vi "MakeToAmbientCode.vi"(4 "ControlInput":string, 10 "AmbientTolerance":dbl=5.0, 11 "TAmbient":dbl=20.0 min=0.0 max=30.0) -> (3 "ToAmbient":string="define onecycle (pwm=100 run pwmloop 5A.PID.Setpoint=-131.500000  while(#3C >-129.5){pause 0.2 s}pwm=10 pause 10 min kill pwmloop pwm=0 relays=0 5A.PID.SetPoint=51.0 while(#3C<50.0){pause 0.2 s} pause 10 min)")   [LabVIEW 2024]
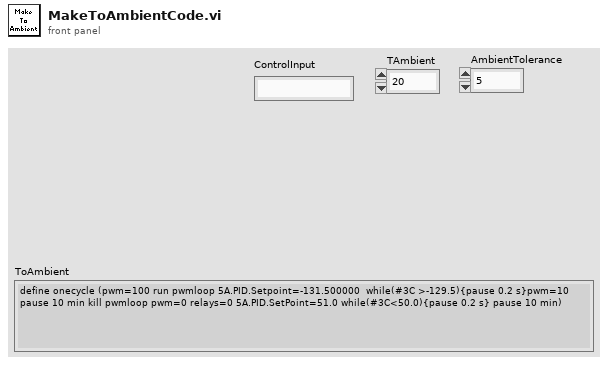
[diagram p1: front panel]
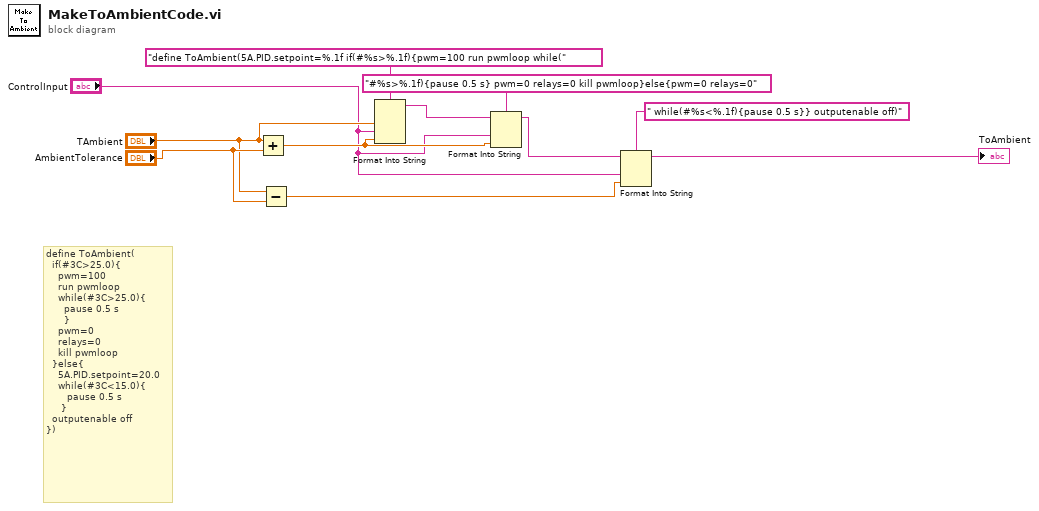
[diagram p0: block diagram]
diagram:
  # "define ToAmbient(\n  if(#3C>25.0){\n    pwm=100 \n    run pwmloop \n    while(#3C>25.0){\n      pause 0.5 s\n      } \n    pwm=0\n    relays=0 \n    kill pwmloop\n  }else{\n    5A.PID.setpoint=20.0 \n    while(#3C<15.0){\n       pause 0.5 s\n     } \n  outputenable off\n})"
  n1 = Add(x="TAmbient", y="AmbientTolerance") -> (x+y=w2:dbl)
  n2 = Subtract(x="TAmbient", y="AmbientTolerance") -> (x-y=w4:dbl)
  n3 = Format Into String(format string="define ToAmbient(5A.PID.setpoint=%.1f if(#%s>%.1f){pwm=100 run pwmloop while(", "TAmbient", "ControlInput", w2) -> (resulting string=w10:string)  [unwired: 2 in, 1 out]
  n4 = Format Into String(format string="#%s>%.1f){pause 0.5 s} pwm=0 relays=0 kill pwmloop}else{pwm=0 relays=0", initial string=w10, "ControlInput", w2) -> (resulting string=w7:string)  [unwired: 1 in, 1 out]
  n5 = Format Into String(format string=" while(#%s<%.1f){pause 0.5 s}} outputenable off)", initial string=w7, "ControlInput", w4) -> (resulting string=→"ToAmbient":string)  [unwired: 1 in, 1 out]
